vi "check_instr_type.vi"(5 "Error generation (Error if missing)":T1(ring), 7 "Attribute":T2={"Identifier"="", "Descriptive name"="", "Data Type"=enum."Integer 32", "Command"="", "Access"=2, "Range Table"="", "Read Callback"="", "Write Callback"="", "Range Callback"="", "Check Callback"="", "Rngtable Callback"="", "Coerce Callback"="", "Supported Models"="", "Instrument Options"="", "Repeated Capabilities"="", "Check Status Callback"="", "Index"=0, "Flag: OPC Wait"=FALSE, "Flag: Dont check status"=FALSE, "Flag: Cache Only"=FALSE} {"Access" items=["Read Only", "Write Only", "Read/Write"]}, 8 "error in":errorcluster, 11 "VISA resource name":refnum<visa-resource-name>) -> (0 "error out":errorcluster, 2 "Instrument present":bool, 3 "VISA resource name out":refnum<visa-resource-name>)   [LabVIEW 2014, in "rszvl_rsidr_core.lvlib"]
uses:
  rszvl_rsidr_core.lvlib
  type_Attribute.ctl
  type_Attribute_Data_Type.ctl
  type_Error_Codes.ctl
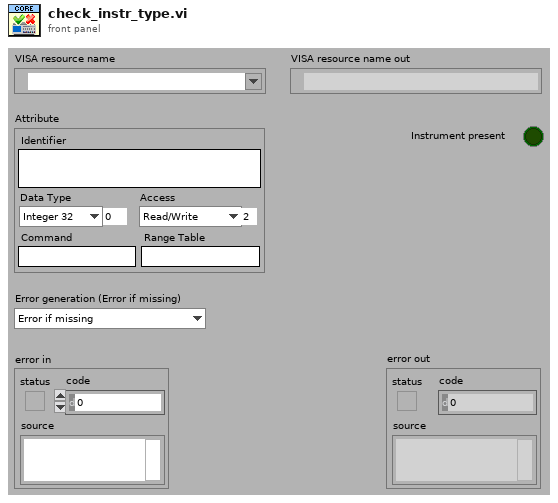
[diagram p1: front panel]
types:
  T1 = enum16{"Error if missing", "Error if present", "No error"}
  T2 = typedef "rszvl_rsidr_core.lvlib/type_Attribute.ctl" = cluster{"Identifier":string, "Descriptive name":string, "Data Type":T3, "Command":string, "Access":u16, "Range Table":string, "Read Callback":string, "Write Callback":string, "Range Callback":string, "Check Callback":string, "Rngtable Callback":string, "Coerce Callback":string, "Supported Models":string, "Instrument Options":string, "Repeated Capabilities":string, "Check Status Callback":string, "Index":i32, "Flag: OPC Wait":bool, "Flag: Dont check status":bool, "Flag: Cache Only":bool}
  T3 = typedef "rszvl_rsidr_core.lvlib/type_Attribute_Data_Type.ctl" = enum16{"Integer 32", "Double", "String", "Boolean", "None", "Integer 64"}
  T4 = typedef "rszvl_rsidr_core.lvlib/type_Error_Codes.ctl" = enum16{"No_error", "VISA_err_ResourceNotFound", "VISA_err_Timeout", "VISA_warn_MoreDataAvailable", "RS_err_MissingCallback", "RS_err_InvalidAttribute", "RS_err_InvalidValue", "RS_err_UnknownResource", "RS_err_AlreadyInitialized", "RS_err_InstrumentStatus", "RS_err_BadRepCapName", "RS_err_TypesMismatch", "RS_err_ValueNotSupported", "RS_err_InvalidRngTable", "RS_err_IDqueryFail", "RS_err_UnexpResponse", "VISA_warn_ConfigNotLoaded", "RS_err_AttributeNotReadable", "RS_err_AttributeNotWritable", "RS_err_InstrumentType", "RS_err_InstrumentOption", "VISA_err_InvalidSize", "RS_err_ReliabilityIndicator", "VISA_warn_UnknownStatus", "VISA_warn_TermCharRead", "VISA_err_IO_error"}
  T5 = typedef "rszvl_rsidr_core.lvlib/type_Session_Data.ctl" = cluster{"Instr type":string, "Instr type for err. msg.":string, "Installed Options":string[], "OPC Timeout":i32, "Query Instrument Status":bool, "Check Range":bool, "Check Options":bool, "Add LF to Write":bool, "Simulate":bool, "Logging":bool, "Logging params":variant, "Interface Type":enum16{"Unknown", "GPIB", "VXI", "GPIB_VXI", "ASRL", "PXI", "TCPIP", "USB", "SOCKET"}, "Fast Sweep":i32, "AdditionalFlags":i32, "WaitBeforeWrite":i32, "WaitBeforeRead":i32, "BinDataChunkSize":i64}
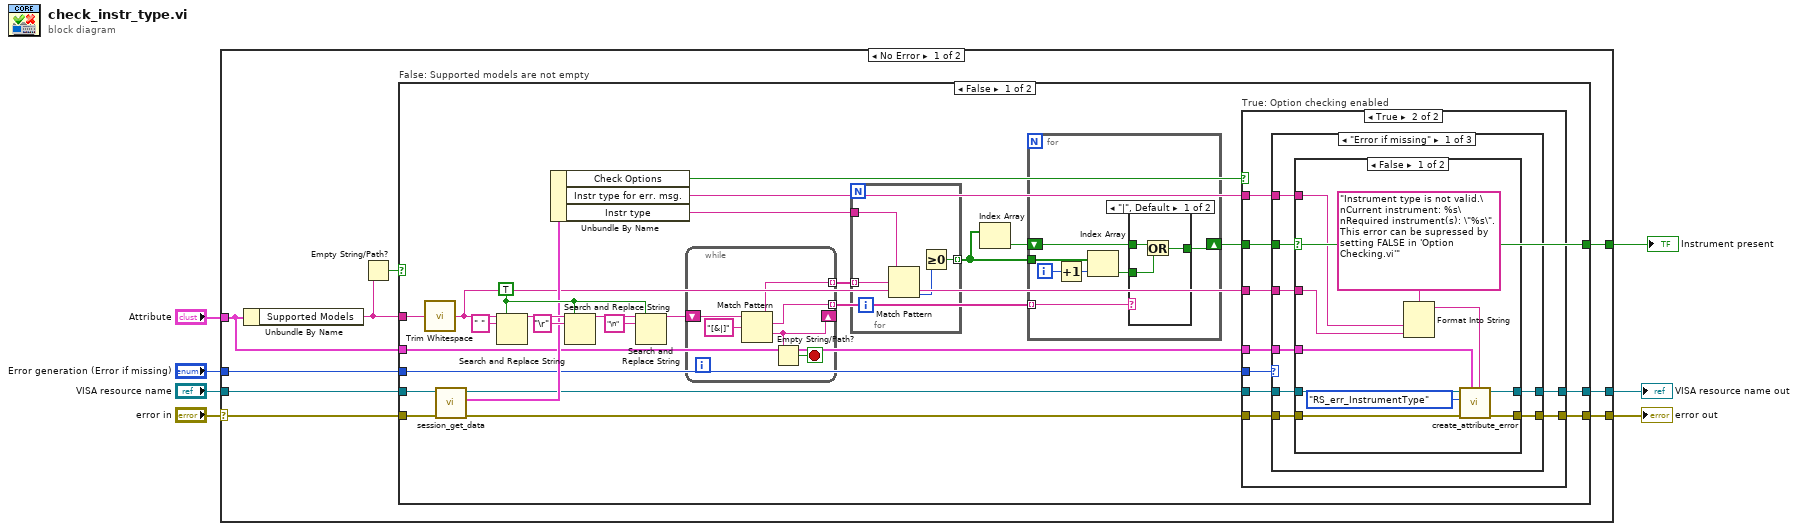
[diagram p0: block diagram]
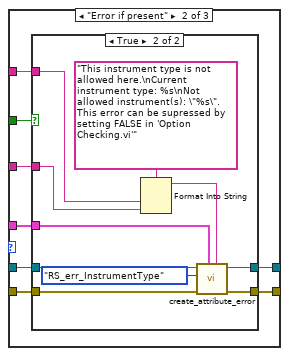
[diagram p4: hidden frame]
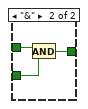
[diagram p7: hidden frame]
diagram:
  n1 = case shown="No Error" "error in" {
    selector: "error in" -> [w10 w121]
    tunnel: [w16 w121] -> w7
    tunnel: "Attribute" -> [w13 _]
    tunnel: "VISA resource name" -> [w11 w122]
    tunnel: [w12 w122] -> w4
    tunnel: [w9 _] -> w2
    tunnel: "Error generation (Error if missing)" -> [w8 _]
    frame No Error {
      n2 = Unbundle By Name(w13) -> ("Supported Models"=w14:string)
      n3 = Empty String/Path?(string/path=w14) -> (empty?=w15:bool)
      n4 = case "False: Supported models are not empty" shown="False" w15 {
        tunnel: w10 -> [w29 w120]
        tunnel: [w22 w120] -> w16
        tunnel: w14 -> [w42 _]
        tunnel: w13 -> [w25 _]
        tunnel: [w19 w119] -> w12
        tunnel: w11 -> [w30 w119]
        tunnel: [w27 _] -> w9
        tunnel: w8 -> [w18 _]
        frame False {
          w32 = TRUE ("replace all? (F)")
          n5 = call "Trim Whitespace.vi"("string"=w42) -> ("trimmed string"=w24:string)  [unwired: 1 in]
          n6 = call "session_get_data.vi"("error in"=w29, "VISA resource name"=w30) -> ("error out"=w23:errorcluster, "Session User Data out"=w28:T5, "VISA resource name out"=w20:refnum<visa-resource-name>)  [unwired: 7 in]
          n7 = Search and Replace String(replace all?=w32, input string=w24, search string=" ") -> (result string=w35:string)  [unwired: 5 in, 3 out]
          n8 = Unbundle By Name(w28) -> ("Check Options"=w21:bool, "Instr type for err. msg."=w26:string, "Instr type"=w17:string)
          n9 = Search and Replace String(replace all?=w32, input string=w35, search string="\r") -> (result string=w34:string)  [unwired: 5 in, 3 out]
          n10 = Search and Replace String(replace all?=w32, input string=w34, search string="\n") -> (result string=w33:string)  [unwired: 5 in, 3 out]
          n11 = while {
            shift-right: [w113] -> _
            shift-left: w33 -> [w118]
            tunnel: [w116] -> w31 mode=indexing
            tunnel: [w115] -> w40 mode=indexing
            stop <- w114 stop-if-true
            n12 = Match Pattern(string=w118, regular expression="[&|]") -> (before substring=w116:string, match substring=w115:string, after substring=w113:string)  [unwired: 1 in, 1 out]
            n13 = Empty String/Path?(string/path=w113) -> (empty?=w114:bool)
          }
          n14 = for {
            tunnel: w31 -> [w111] mode=indexing
            tunnel: [w112] -> w38 mode=indexing
            tunnel: w17 -> [w109]
            n15 = Match Pattern(string=w109, regular expression=w111) -> (offset past match=w110:i32)  [unwired: 1 in, 3 out]
            n16 = Greater Or Equal To 0?(x=w110) -> (x >= 0?=w112:bool)
          }
          n17 = Index Array(array=w38) -> (element=w39:bool)  [unwired: 1 in]
          n18 = for {
            tunnel: w40 -> [w97] mode=indexing
            tunnel: w38 -> [w101]
            shift-right: [w96] -> w27
            shift-left: w39 -> [w102]
            i -> [w99]
            n19 = Increment(x=w99) -> (x+1=w100:i32)
            n20 = Index Array(array=w101, index=w100) -> (element=w98:bool)
            n21 = case shown="\"|\", Default" w97 {
              tunnel: w102 -> [w104 w108]
              tunnel: [w105 w107] -> w96
              tunnel: w98 -> [w103 w106]
              frame "|", Default {
                n22 = Or(x=w104, y=w103) -> (x .or. y?=w105:bool)
              }
              frame "&" {
                n23 = And(x=w108, y=w106) -> (x .and. y?=w107:bool)
              }
            }
          }
          n24 = case "True: Option checking enabled" shown="True" w21 {
            tunnel: w18 -> [_ w53]
            tunnel: w27 -> [_ w52]
            tunnel: w26 -> [_ w51]
            tunnel: w25 -> [_ w50]
            tunnel: w24 -> [_ w49]
            tunnel: w23 -> [w44 w48]
            tunnel: [w44 w47] -> w22
            tunnel: w20 -> [w43 w46]
            tunnel: [w43 w45] -> w19
            frame False {
            }
            frame True {
              n25 = case shown="\"Error if missing\"" w53 {
                tunnel: w52 -> [w61 w81 _]
                tunnel: w51 -> [w59 w79 _]
                tunnel: w50 -> [w60 w80 _]
                tunnel: w49 -> [w58 w78 _]
                tunnel: w48 -> [w57 w77 w95]
                tunnel: [w56 w76 w95] -> w47
                tunnel: w46 -> [w55 w75 w94]
                tunnel: [w54 w74 w94] -> w45
                frame "Error if missing" {
                  n26 = case shown="False" w61 {
                    tunnel: w60 -> [w69 _]
                    tunnel: w59 -> [w68 _]
                    tunnel: w58 -> [w67 _]
                    tunnel: w57 -> [w66 w73]
                    tunnel: [w65 w73] -> w56
                    tunnel: w55 -> [w64 w72]
                    tunnel: [w62 w72] -> w54
                    frame False {
                      n27 = Format Into String(format string="Instrument type is not valid.\nCurrent instrument: %s\nRequired instrument(s): \"%s\". This error can be supressed by setting FALSE in 'Option Checking.vi'" ("string"), w68, w67) -> (resulting string=w71:string)  [unwired: 2 in, 1 out]
                      n28 = call "create_attribute_error.vi"("Error Elaboration (\"\")"=w71, "Attribute"=w69, "error in"=w66, "Error Enum in"=type_Error_Codes."RS_err_InstrumentType" ("Error Enum in (from err to recompose)"), "VISA resource name"=w64) -> ("error out"=w65:errorcluster, "VISA resource name out"=w62:refnum<visa-resource-name>)  [unwired: 5 in]
                    }
                    frame True {
                    }
                  }
                }
                frame "Error if present" {
                  n29 = case shown="True" w81 {
                    tunnel: w80 -> [_ w91]
                    tunnel: w79 -> [_ w90]
                    tunnel: w78 -> [_ w89]
                    tunnel: w77 -> [w83 w88]
                    tunnel: [w83 w87] -> w76
                    tunnel: w75 -> [w82 w85]
                    tunnel: [w82 w84] -> w74
                    frame False {
                    }
                    frame True {
                      n30 = Format Into String(format string="This instrument type is not allowed here.\nCurrent instrument type: %s\nNot allowed instrument(s): \"%s\". This error can be supressed by setting FALSE in 'Option Checking.vi'" ("string"), w90, w89) -> (resulting string=w93:string)  [unwired: 2 in, 1 out]
                      n31 = call "create_attribute_error.vi"("Error Elaboration (\"\")"=w93, "Attribute"=w91, "error in"=w88, "Error Enum in"=type_Error_Codes."RS_err_InstrumentType" ("Error Enum in (from err to recompose)"), "VISA resource name"=w85) -> ("error out"=w87:errorcluster, "VISA resource name out"=w84:refnum<visa-resource-name>)  [unwired: 5 in]
                    }
                  }
                }
                frame "No error" {
                }
              }
            }
          }
        }
        frame True {
        }
      }
    }
    frame Error {
    }
  }
  "error out" <- w7
  "VISA resource name out" <- w4
  "Instrument present" <- w2
